vi "Read configuration.vi"(8 "error in":errorcluster, 11 "dds editor node in":refnum<class "DDS editor node.lvclass">) -> (0 "error out":errorcluster, 2 "configuration":refnum<class "NISE_CEF_serializable configuration.lvclass">, 3 "dds editor node out":refnum<class "DDS editor node.lvclass">)   [LabVIEW 2014, in "DDS editor node.lvclass"]
uses:
  DDS editor node.lvclass
  <vilib>/NI/Configuration Framework/serializable configuration/NISE_CEF_serializable configuration.lvclass
  DDS editor node.lvclass/DDS editor node.ctl
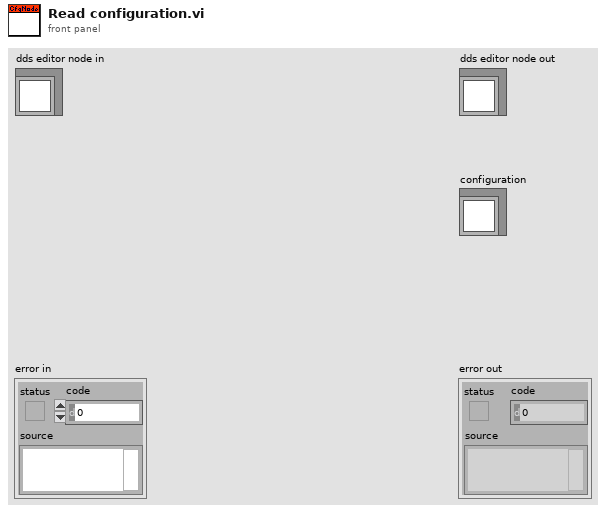
[diagram p1: front panel]
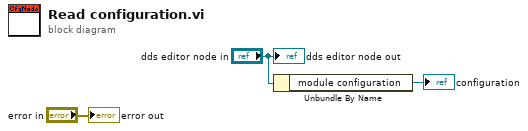
[diagram p0: block diagram]
diagram:
  n1 = Unbundle By Name("dds editor node in") -> ("module configuration"=→"configuration":refnum<class "DDS configuration.lvclass">)
  "error out" <- "error in"
  "dds editor node out" <- "dds editor node in"
